vi "Get Transfer UIs.vi"(8 "error in (no error)":errorcluster, 11 "Component UI in":refnum<class "UDP User Interfaces.lvclass">=refnum) -> (0 "error out":errorcluster, 1 "Tx Transfer UI":refnum<class "User Interface.lvclass">, 2 "Rx Transfer UI":refnum<class "User Interface.lvclass">, 3 "Component UI out":refnum<class "UDP User Interfaces.lvclass">)   [LabVIEW 2020, in "UDP.lvlib" / "UDP User Interfaces.lvclass"]
uses:
  UDP User Interfaces.lvclass
  Transfer Rx/UDP Transfer Rx User Interface.lvclass
  Transfer Tx/UDP Transfer Tx User Interface.lvclass
  DSF Core.lvlibp/Classes/User Interface/User Interface.lvclass
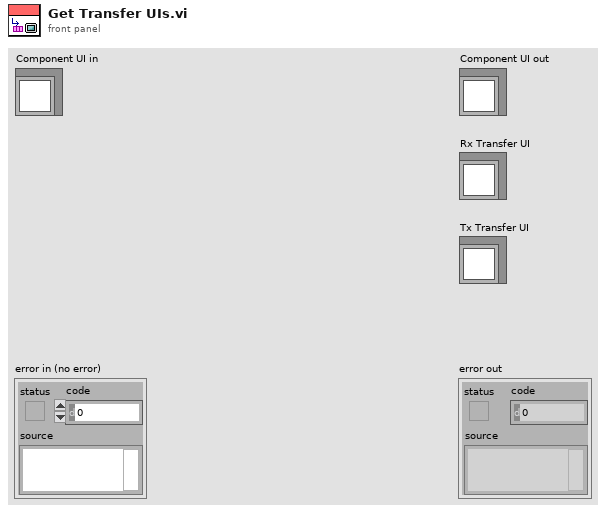
[diagram p1: front panel]
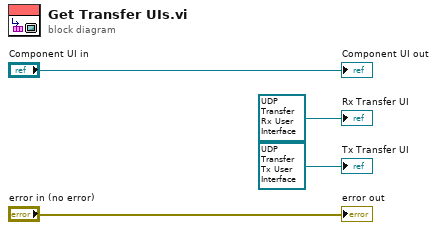
[diagram p0: block diagram]
diagram:
  "error out" <- "error in (no error)"
  "Component UI out" <- "Component UI in"
  "Rx Transfer UI" <- refnum<class "UDP Transfer Rx User Interface.lvclass"> refnum ("UDP Transceiver.lvlib:UDP Transfer Rx User Interface.lvclass")
  "Tx Transfer UI" <- refnum<class "UDP Transfer Tx User Interface.lvclass"> refnum ("UDP Transceiver.lvlib:UDP Transfer Tx User Interface.lvclass")
